vi "Scale Regression.vi"(8 "error in (no error)":errorcluster, 9 "Read CSV":bool, 10 "TScale Calibration":dbl[][](array[numeric]), 11 "GUI in":refnum<class "GUI.lvclass">) -> (0 "error out":errorcluster, 3 "GUI out":refnum<class "GUI.lvclass">)   [LabVIEW 2020, in "GUI.lvlib" / "GUI.lvclass"]
uses:
  GUI.lvclass
  GUI.lvclass/GUI.ctl
  <vilib>/Utility/file.llb/Write Delimited Spreadsheet (DBL).vi
  <vilib>/Utility/file.llb/Read Delimited Spreadsheet (DBL).vi
  <vilib>/Analysis/NI_AALPro.lvlib
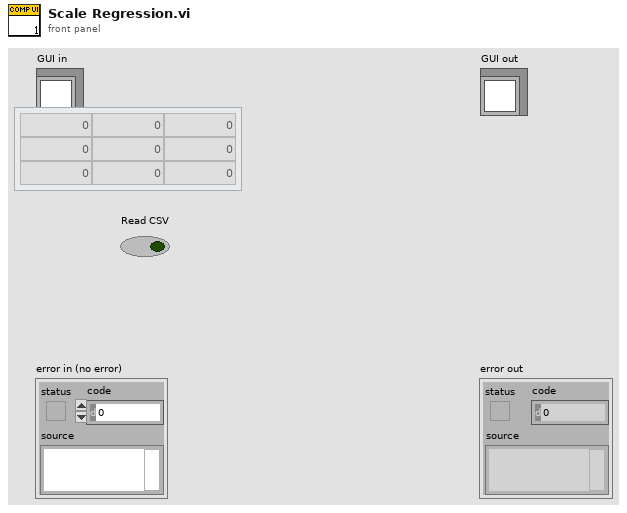
[diagram p1: front panel]
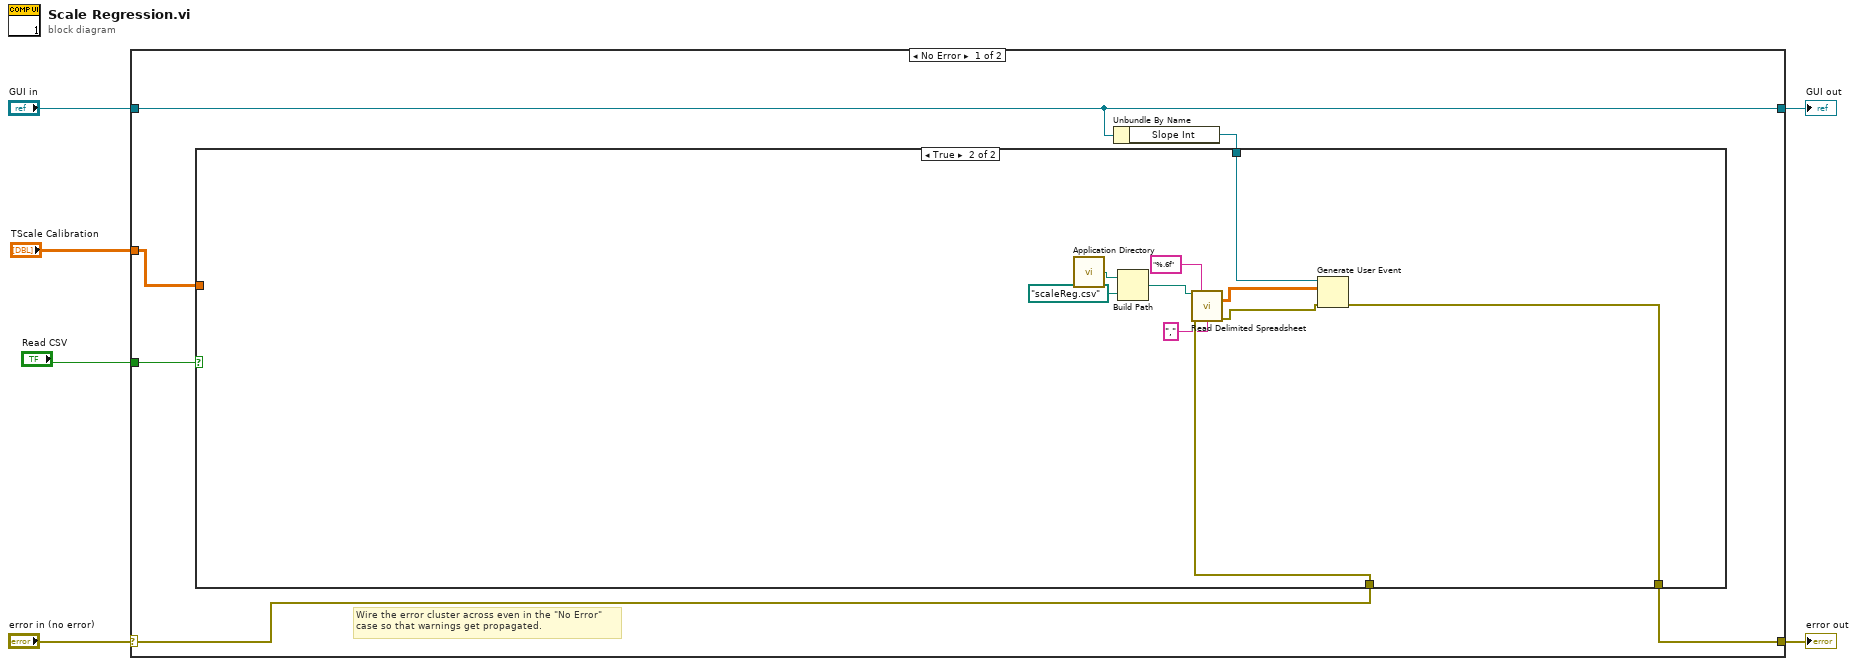
[diagram p0: block diagram]
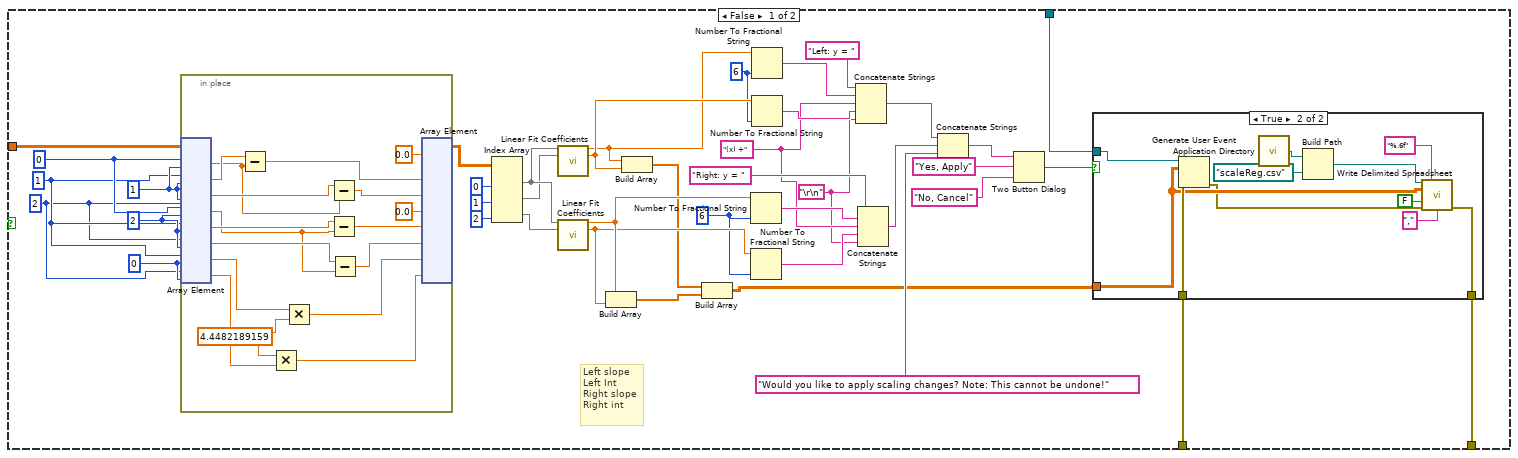
[diagram p2: hidden frame]
diagram:
  n1 = case shown="No Error" "error in (no error)" {
    selector: "error in (no error)" -> [w8 w94]
    tunnel: [w9 w94] -> w5
    tunnel: [w11 w93] -> w3
    tunnel: "GUI in" -> [w11 w93]
    tunnel: "TScale Calibration" -> [w12 _]
    tunnel: "Read CSV" -> [w7 _]
    frame No Error {
      # "Wire the error cluster across even in the \"No Error\"\ncase so that warnings get propagated."
      n2 = Unbundle By Name(w11) -> ("Slope Int"=w10:refnum<user-event>)
      n3 = case shown="True" w7 {
        tunnel: w12 -> [w53 _]
        tunnel: w10 -> [w22 w89]
        tunnel: [w16 w85] -> w9
        tunnel: w8 -> [w15 w86]
        frame False {
          w13 = i16 6 ("width (-)")
          w14 = i16 6 ("width (-)")
          w30 = "\r\n"
          w32 = "(x) +" ("string")
          w45 = 0
          w51 = 2
          w43 = 2
          w44 = 1
          w46 = 0
          w52 = 1
          # "Left slope\nLeft Int\nRight slope\nRight int"
          n4 = in-place {
            w68 = 4.4482189159 ("x")
            n5 = in-place-array #1(w53, w46, w52, w44, w52, w43, w52, w46, w51, w44, w51, w43, w51, w44, w45, w43, w45) -> (w77:dbl, w80:dbl, w78:dbl, w73:dbl, w75:dbl, w74:dbl, w70:dbl, w69:dbl)
            n6 = Subtract(x=w80, y=w77) -> (x-y=w79:dbl)
            n7 = Multiply(x=w68, y=w69) -> (x*y=w66:dbl)
            n8 = Multiply(x=w70, y=w68) -> (x*y=w67:dbl)
            n9 = Subtract(x=w78, y=w77) -> (x-y=w76:dbl)
            n10 = Subtract(x=w75, y=w73) -> (x-y=w72:dbl)
            n11 = Subtract(x=w74, y=w73) -> (x-y=w71:dbl)
            n12 = in-place-array #1(0.0 ("element"), w79, w76, 0.0 ("element"), w72, w71, w67, w66) -> (w50:dbl[][])  [unwired: 16 out]
          }
          n13 = Index Array(array=w50, index (col) #1=0 ("disabled index (col)"), index (col) #2=1 ("index (col)"), index (col) #3=2 ("index (col)")) -> (element #1=w42:dbl[], element #2=w41:dbl[], element #3=w40:dbl[])  [unwired: 3 in]
          n14 = call <vilib>:"Linear Fit Coefficients.vi"("Y"=w42, "X"=w41) -> ("slope"=w38:dbl, "intercept"=w39:dbl)  [unwired: 11 in, 1 out]
          n15 = call <vilib>:"Linear Fit Coefficients.vi"("Y"=w42, "X"=w40) -> ("slope"=w21:dbl, "intercept"=w20:dbl)  [unwired: 11 in, 1 out]
          n16 = Build Array(w21, w20) -> (w18:dbl[])
          n17 = Build Array(w38, w39) -> (w19:dbl[])
          n18 = Build Array(w19, w18) -> (w17:dbl[][])
          n19 = Number To Fractional String(number=w21, precision (6)=w13) -> (F-format string=w33:string)  [unwired: 2 in]
          n20 = Number To Fractional String(number=w20, precision (6)=w13) -> (F-format string=w31:string)  [unwired: 2 in]
          n21 = Number To Fractional String(number=w38, precision (6)=w14) -> (F-format string=w36:string)  [unwired: 2 in]
          n22 = Number To Fractional String(number=w39, precision (6)=w14) -> (F-format string=w35:string)  [unwired: 2 in]
          n23 = Concatenate Strings("Left: y = " ("string"), w36, w32, w35, w30) -> (w29:string)
          n24 = Concatenate Strings("Right: y = " ("string"), w33, w32, w31, w30) -> (w28:string)
          n25 = Concatenate Strings(w29, w28, "Would you like to apply scaling changes? Note: This cannot be undone!" ("string")) -> (w26:string)
          n26 = Two Button Dialog(message=w26, 1:"No, Cancel" ("F button name (\"Cancel\")"), 2:"Yes, Apply" ("T button name (\"OK\")")) -> (T button?=w23:bool)
          n27 = case shown="True" w23 {
            tunnel: w22 -> [_ w65]
            tunnel: w17 -> [_ w61]
            tunnel: [w54 w55] -> w16
            tunnel: w15 -> [w54 w64]
            frame False {
            }
            frame True {
              n28 = Generate User Event(user event=w65, event data cluster=w61, error in=w64) -> (error out=w60:errorcluster)  [unwired: 1 in, 1 out]
              n29 = call <vilib>:"Application Directory.vi"() -> ("Application Directory"=w63:path)
              n30 = Build Path(base path=w63, name or relative path=path "scaleReg.csv") -> (appended path=w62:path)
              n31 = call-poly <vilib>:"Write Delimited Spreadsheet.vi"("file path (dialog if empty)"=w62, "format (%.3f)"="%.6f", "2D data"=w61, "append to file? (new file:F)"=FALSE, "error in (no error)"=w60, "delimiter (\\t)"="," ("delimiter (\\t)")) -> ("error out"=w55:errorcluster)  [unwired: 8 in, 1 out]
            }
          }
        }
        frame True {
          n32 = call <vilib>:"Application Directory.vi"() -> ("Application Directory"=w92:path)
          n33 = Build Path(base path=w92, name or relative path=path "scaleReg.csv") -> (appended path=w90:path)
          n34 = call-poly <vilib>:"Read Delimited Spreadsheet.vi"("file path (dialog if empty)"=w90, "format (%.3f)"="%.6f", "error in (no error)"=w86, "delimiter (\\t)"="," ("delimiter (\\t)")) -> ("all rows"=w88:dbl[][], "error out"=w87:errorcluster)  [unwired: 6 in, 4 out]
          n35 = Generate User Event(user event=w89, event data cluster=w88, error in=w87) -> (error out=w85:errorcluster)  [unwired: 1 in, 1 out]
        }
      }
    }
    frame Error {
    }
  }
  "error out" <- w5
  "GUI out" <- w3
